vi "create.OrderExecuted.vi"(8 "error in (no error)":errorcluster, 10 "OrderExecuted.Parms":T1={"Time Offset"=457000, "Order Id"="ORID0001", "Executed\nQuantity"=200, "Execution Id"=0}, 11 "OrderExecuted in":refnum<class "OrderExecuted.lvclass">) -> (0 "error out":errorcluster, 3 "OrderExecuted out":refnum<class "OrderExecuted.lvclass">)   [LabVIEW 2022 SP3, in "OrderExecuted.lvclass"]
uses:
  OrderExecuted.lvclass
  OrderExecuted.Parameters.ctl
  FieldSpec.ctl
  PitchMessage/FieldValue.ctl
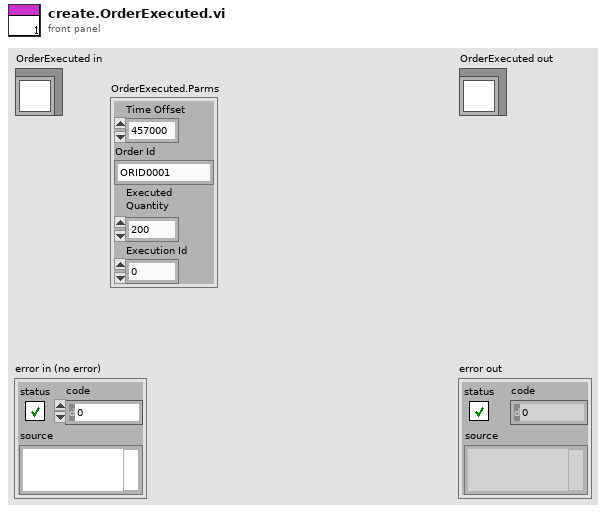
[diagram p1: front panel]
types:
  T1 = typedef "OrderExecuted.lvclass/OrderExecuted.Parameters.ctl" = cluster{"Time Offset":u32, "Order Id":string, "Executed\nQuantity":u32, "Execution Id":u64}
  T2 = typedef "FieldSpec.ctl" = cluster{"Name":string, "Offset":i32, "Length":i32, "FieldType":enum16{"Alphanumeric", "Binary", "BinaryLongPrice", "BinaryShortPrice", "BitField", "PrintableAscii", "Value"}}
  T3 = typedef "FieldValue.ctl" = variant
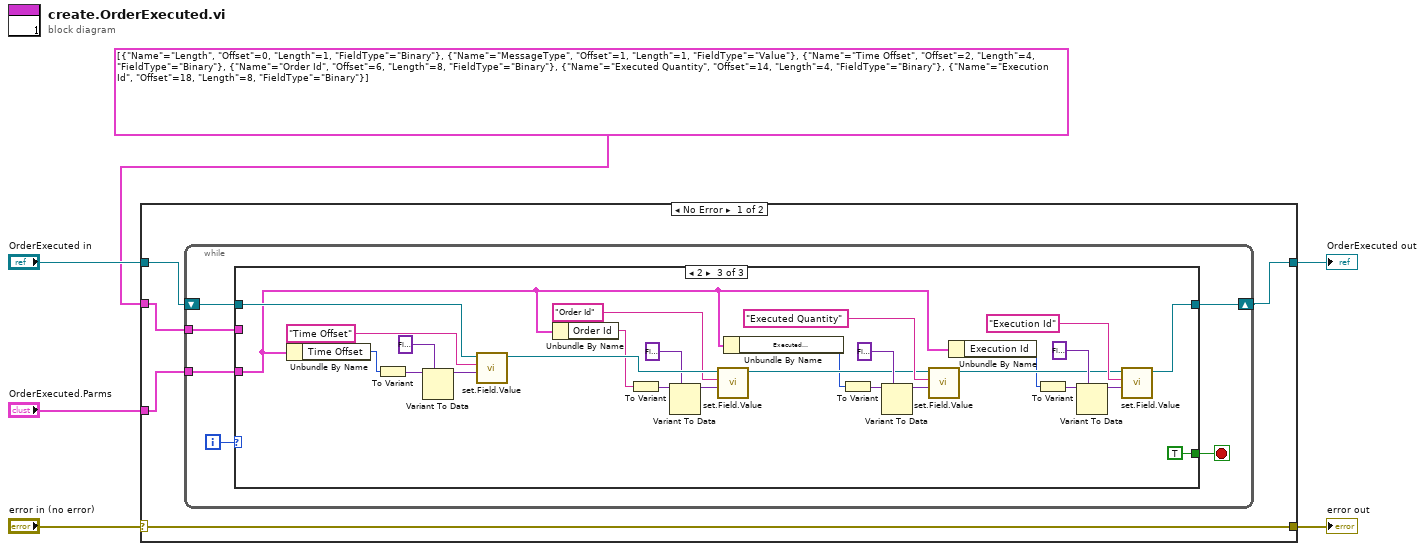
[diagram p0: block diagram]
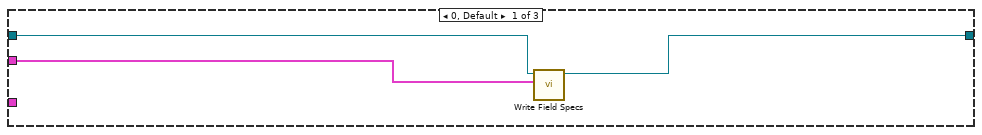
[diagram p2: hidden frame]
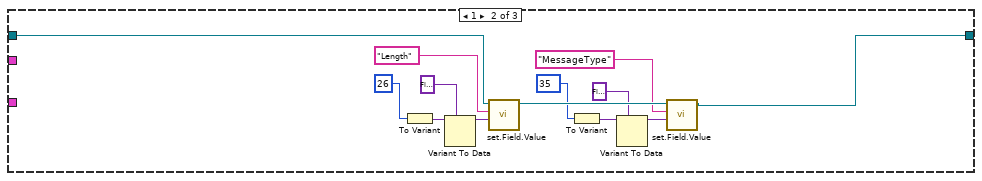
[diagram p3: hidden frame]
diagram:
  n1 = case shown="No Error" "error in (no error)" {
    selector: "error in (no error)" -> [w11 w62]
    tunnel: [w11 w62] -> w5
    tunnel: [w7 w61] -> w3
    tunnel: "OrderExecuted in" -> [w10 w61]
    tunnel: T2[] [{"Name"="Length", "Offset"=0, "Length"=1, "FieldType"=enum."Binary"}, {"Name"="MessageType", "Offset"=1, "Length"=1, "FieldType"=enum."Value"}, {"Name"="Time Offset", "Offset"=2, "Length"=4, "FieldType"=enum."Binary"}, {"Name"="Order Id", "Offset"=6, "Length"=8, "FieldType"=enum."Binary"}, {"Name"="Executed Quantity", "Offset"=14, "Length"=4, "FieldType"=enum."Binary"}, {"Name"="Execution Id", "Offset"=18, "Length"=8, "FieldType"=enum."Binary"}] ("appended array") -> [w9 _]
    tunnel: "OrderExecuted.Parms" -> [w8 _]
    frame No Error {
      n2 = while {
        tunnel: w9 -> [w16]
        shift-right: [w14] -> w7
        shift-left: w10 -> [w15]
        tunnel: w8 -> [w12]
        i -> [w17]
        stop <- w13 stop-if-true
        n3 = case shown="2" w17 {
          tunnel: [_ _ TRUE] -> w13
          tunnel: w16 -> [w20 _ _]
          tunnel: w15 -> [w19 w22 w51]
          tunnel: [w18 w21 w40] -> w14
          tunnel: w12 -> [_ _ w36]
          frame 0, Default {
            n4 = call-dynamic "Write Field Specs.vi"("Field Specs"=w20, "PitchMessage in"=w19) -> ("PitchMessage out"=w18:refnum<class "OrderExecuted.lvclass">)  [unwired: 8 in, 1 out]
          }
          frame 1 {
            n5 = To Variant(anything=u8 26 ("Value")) -> (Variant=w29:variant)
            n6 = Variant To Data(type=T3 variant ("FieldValue"), Variant=w29) -> (data=w30:T3)  [unwired: 1 in, 1 out]
            n7 = call-dynamic "set.Field.Value.vi"("Value"=w30, "FIeld.Name"="Length", "PitchMessage in"=w22) -> ("PitchMessage out"=w31:refnum<class "OrderExecuted.lvclass">)  [unwired: 7 in, 1 out]
            n8 = To Variant(anything=u8 35 ("Value")) -> (Variant=w32:variant)
            n9 = Variant To Data(type=T3 variant ("FieldValue"), Variant=w32) -> (data=w33:T3)  [unwired: 1 in, 1 out]
            n10 = call-dynamic "set.Field.Value.vi"("Value"=w33, "FIeld.Name"="MessageType", "PitchMessage in"=w31) -> ("PitchMessage out"=w21:refnum<class "OrderExecuted.lvclass">)  [unwired: 7 in, 1 out]
          }
          frame 2 {
            n11 = Unbundle By Name(w36) -> ("Time Offset"=w39:u32)
            n12 = To Variant(anything=w39) -> (Variant=w56:variant)
            n13 = Variant To Data(type=T3 variant ("FieldValue"), Variant=w56) -> (data=w57:T3)  [unwired: 1 in, 1 out]
            n14 = call-dynamic "set.Field.Value.vi"("Value"=w57, "FIeld.Name"="Time Offset", "PitchMessage in"=w51) -> ("PitchMessage out"=w59:refnum<class "OrderExecuted.lvclass">)  [unwired: 7 in, 1 out]
            n15 = Unbundle By Name(w36) -> ("Order Id"=w38:string)
            n16 = To Variant(anything=w38) -> (Variant=w58:variant)
            n17 = Variant To Data(type=T3 variant ("FieldValue"), Variant=w58) -> (data=w60:T3)  [unwired: 1 in, 1 out]
            n18 = call-dynamic "set.Field.Value.vi"("Value"=w60, "FIeld.Name"="Order Id", "PitchMessage in"=w59) -> ("PitchMessage out"=w46:refnum<class "OrderExecuted.lvclass">)  [unwired: 7 in, 1 out]
            n19 = Unbundle By Name(w36) -> ("Executed\nQuantity"=w37:u32)
            n20 = To Variant(anything=w37) -> (Variant=w49:variant)
            n21 = Variant To Data(type=T3 variant ("FieldValue"), Variant=w49) -> (data=w50:T3)  [unwired: 1 in, 1 out]
            n22 = call-dynamic "set.Field.Value.vi"("Value"=w50, "FIeld.Name"="Executed Quantity", "PitchMessage in"=w46) -> ("PitchMessage out"=w41:refnum<class "OrderExecuted.lvclass">)  [unwired: 7 in, 1 out]
            n23 = Unbundle By Name(w36) -> ("Execution Id"=w35:u64)
            n24 = To Variant(anything=w35) -> (Variant=w44:variant)
            n25 = Variant To Data(type=T3 variant ("FieldValue"), Variant=w44) -> (data=w45:T3)  [unwired: 1 in, 1 out]
            n26 = call-dynamic "set.Field.Value.vi"("Value"=w45, "FIeld.Name"="Execution Id", "PitchMessage in"=w41) -> ("PitchMessage out"=w40:refnum<class "OrderExecuted.lvclass">)  [unwired: 7 in, 1 out]
          }
        }
      }
    }
    frame Error {
    }
  }
  "error out" <- w5
  "OrderExecuted out" <- w3
